vi "HEX强制转换.vi"(1 "HexString":string) -> (0 "HEX":string)   [LabVIEW 2020]
panel:
  # "本VI的作用是将以字符串形式输入的HEX转化为HEX\n例如:\n输入字符串:FFFFAAAA（字符串格式）\n转化为HEX:FFFFAAAA（HEX格式）"
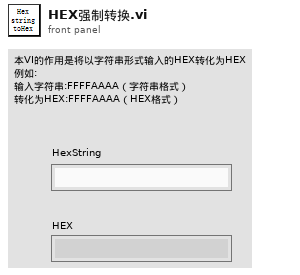
[diagram p1: front panel]
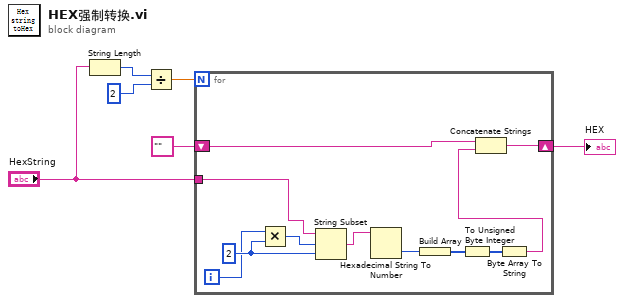
[diagram p0: block diagram]
diagram:
  n1 = String Length(string="HexString") -> (length=w5:i32)
  n2 = Divide(x=w5, y=2) -> (x/y=w1:dbl)
  n3 = for {
    N: w1 -> [_]
    tunnel: "HexString" -> [w14]
    shift-right: [w17] -> w2
    shift-left: "" -> [w8]
    i -> [w7]
    w16 = 2
    n4 = Multiply(x=w7, y=w16) -> (x*y=w15:i32)
    n5 = String Subset(string=w14, offset (0)=w15, length (rest)=w16) -> (substring=w13:string)
    n6 = Hexadecimal String To Number(string=w13) -> (number=w12:u32)  [unwired: 2 in, 1 out]
    n7 = Build Array(w12) -> (w11:u32[])
    n8 = To Unsigned Byte Integer(number=w11) -> (unsigned 8bit integer=w10:u8[])
    n9 = Byte Array To String(unsigned byte array=w10) -> (string=w9:string)
    n10 = Concatenate Strings(w8, w9) -> (w17:string)
  }
  "HEX" <- w2
